vi "Up-Down.vi"(10 "Down":bool, 11 "Up":bool) -> (2 "Direction":dbl)   [LabVIEW 2014]
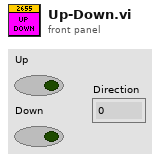
[diagram p1: front panel]
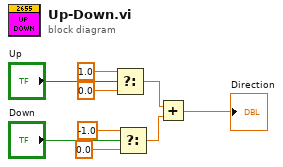
[diagram p0: block diagram]
diagram:
  n1 = Select(t=1.0, s="Up", f=0.0) -> (s? t:f=w5:dbl)
  n2 = Select(t=-1.0, s="Down", f=0.0) -> (s? t:f=w4:dbl)
  n3 = Add(x=w5, y=w4) -> (x+y=→"Direction":dbl)
